vi "Problem 16 - Power digit sum.vi"() -> (3 "Answer (sum of digits)":i32)   [LabVIEW 2021, in "Project Euler.lvlib"]
uses:
  Project Euler.lvlib
  Utilities/Named Timers/Named Timers.lvlib
  Utilities/Numeric Utilities/Numeric Utilities.lvlib
panel:
  out "no. of characters":i32
  out "Loop iteration":i32
  out "2^n":string
  in  "n":i32=1000
  out "Total execution time (ms)":u32
  # "Development\nControls or indicators that are useful for development or testing, but which are not outputs of the VI."
  # "Input\nInputs to the VI"
  # "Output\nOutputs of the VI"
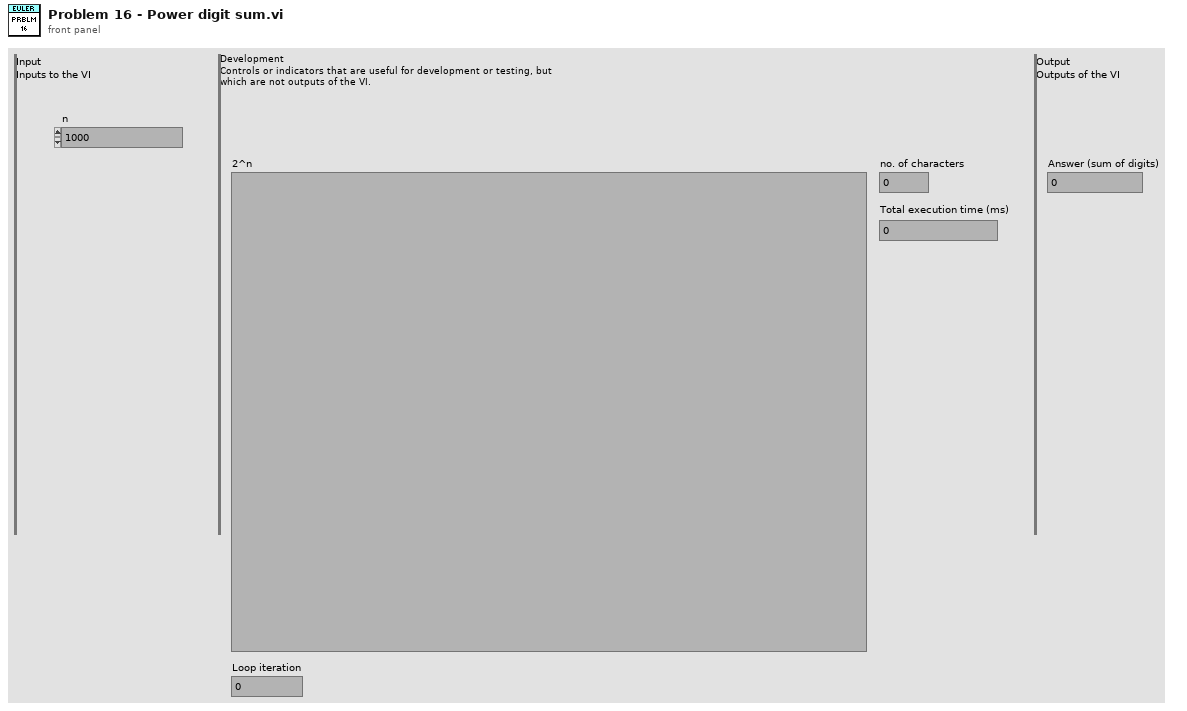
[diagram p1: front panel]
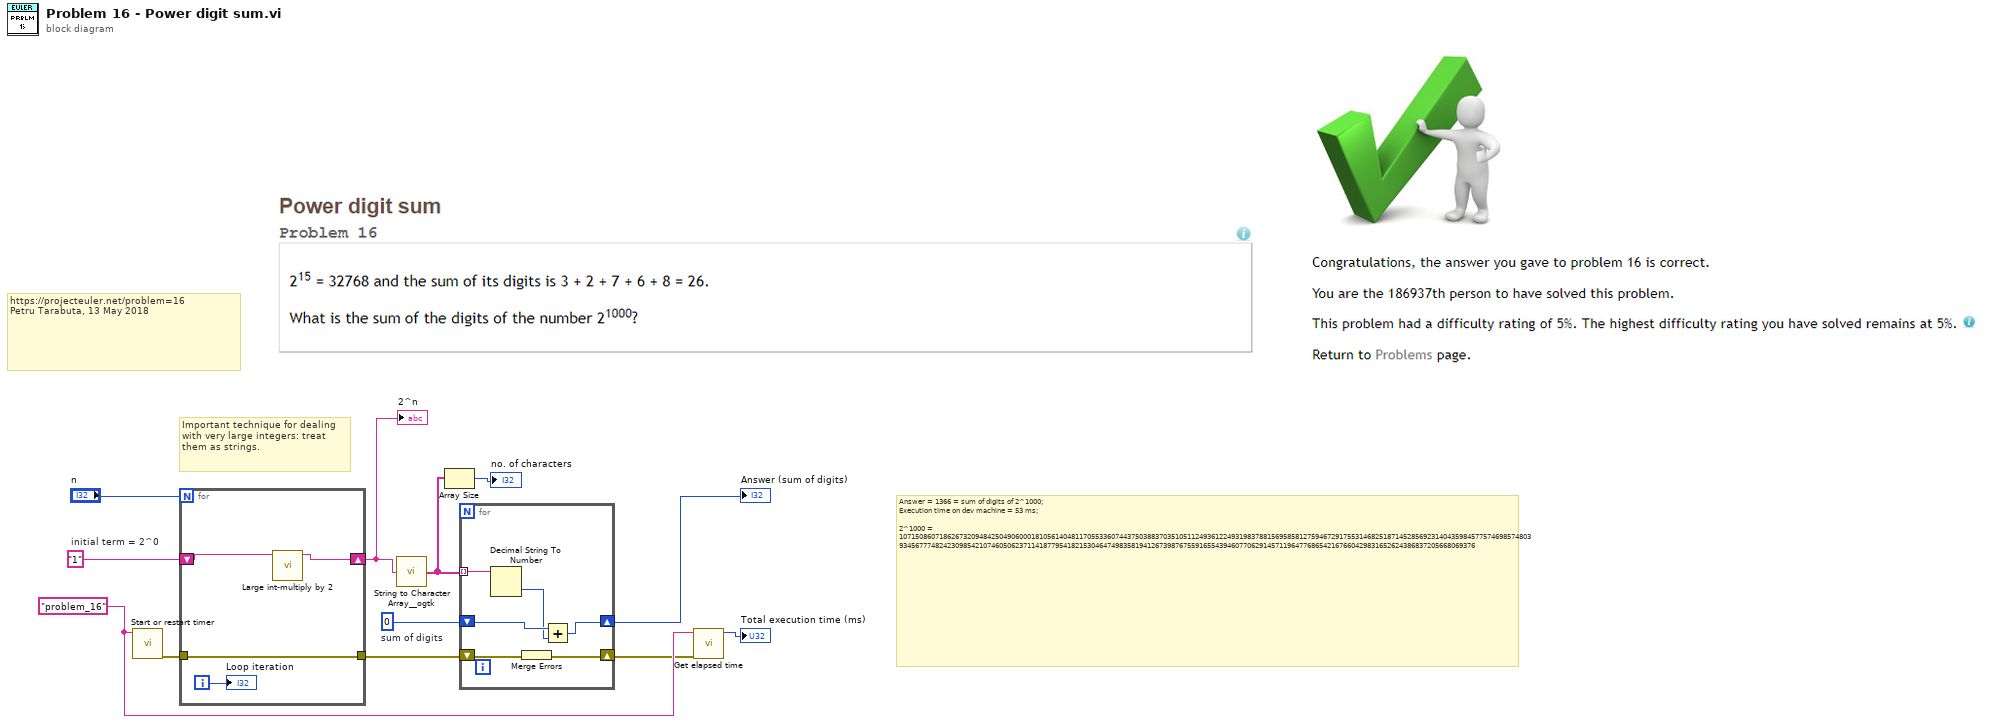
[diagram p0: block diagram]
diagram:
  w4 = 0  # sum of digits
  w11 = "1"  # initial term = 2^0
  w7 = "problem_16" ("Timer name")
  # "Important technique for dealing with very large integers: treat them as strings."
  # "Answer = 1366 = sum of digits of 2^1000;\nExecution time on dev machine = 53 ms;\n\n2^1000 = 10715086071862673209484250490600018105614048117055336074437503883703510511249361224931983788156958581275946729175531468251871452856923140435984577574698574803934567774824230985421074605062371141877954182153046474983581941267398767559165543946077062914571196477686542167660429831652624386837205668069376"
  # "https://projecteuler.net/problem=16\nPetru Tarabuta, 13 May 2018"
  n1 = call "Start or restart timer.vi"("Timer name"=w7) -> ("error out"=w9:errorcluster)  [unwired: 10 in]
  n2 = for {
    N: "n" -> [_]
    shift-right: [w15] -> w6
    shift-left: w11 -> [w16]
    tunnel: w9 -> [w14]
    tunnel: [w14] -> w8
    i -> [w13]
    n3 = call "Large int-multiply by 2.vi"("Large int (decimal)"=w16) -> ("Large int (multiplied by 2)"=w15:string)  [unwired: 8 in, 2 out]
    "Loop iteration" <- w13
  }
  "2^n" <- w6
  n4 = call <userlib>:"String to Character Array__ogtk.vi"("Input String"=w6) -> ("Character Array"=w2:string[])
  n5 = Array Size(array=w2) -> (size(s)=→"no. of characters":i32)
  n6 = for {
    shift-right: [w21] -> w5
    shift-left: w8 -> [w22]
    tunnel: w2 -> [w20] mode=indexing
    shift-right: [w17] -> w3
    shift-left: w4 -> [w19]
    n7 = Decimal String To Number(string=w20) -> (number=w18:i32)  [unwired: 2 in, 1 out]
    n8 = Merge Errors(w22) -> (w21:errorcluster)
    n9 = Add(x=w19, y=w18) -> (x+y=w17:i32)
  }
  "Answer (sum of digits)" <- w3
  n10 = call "Get elapsed time.vi"("error in (no error)"=w5, "Timer name"=w7) -> ("Elapsed time (ms)"=→"Total execution time (ms)":u32)  [unwired: 6 in, 3 out]
